vi "Test Get Documentation.vi"(8 "error in (no error)":errorcluster, 11 "Test Template in":refnum<class "niDTS BT Rx Test.lvclass">) -> (0 "error out":errorcluster, 2 "Documentation":T1, 3 "Test Template out":refnum<class "niDTS BT Rx Test.lvclass">)   [LabVIEW 2015, in "niDTS BT.lvlib" / "niDTS BT Rx Test.lvclass"]
uses:
  niDTS BT Rx Test.lvclass
  Framework/Test/Includes/niDTS Test INC Documentation.ctl
  Framework/niDTS Framework.lvlib
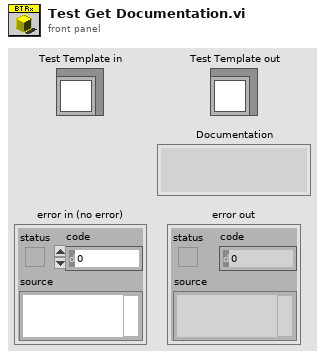
[diagram p1: front panel]
types:
  T1 = typedef "niDTS Framework.lvlib/niDTS Test INC Documentation.ctl" = string
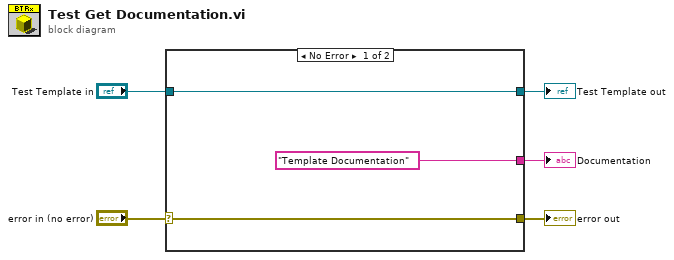
[diagram p0: block diagram]
diagram:
  n1 = case shown="No Error" "error in (no error)" {
    selector: "error in (no error)" -> [w7 w10]
    tunnel: [w7 w10] -> w4
    tunnel: [w8 w9] -> w2
    tunnel: "Test Template in" -> [w8 w9]
    tunnel: [T1 "Template Documentation" ("Documentation") _] -> w1
    frame No Error {
    }
    frame Error {
    }
  }
  "error out" <- w4
  "Test Template out" <- w2
  "Documentation" <- w1
